vi "AM Measurement Compensation.vi"(11 "Mean Data in":dbl[](array[numeric])) -> (3 "Mean Data Compensated out":dbl[](array[numeric]))   [LabVIEW 2020, in "Motion.lvlib"]
uses:
  Motion.lvlib
  support/PCT FGV CMD.ctl
  Test Driver/Test Driver.lvlib
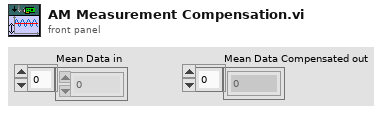
[diagram p1: front panel]
types:
  T1 = typedef "PCT FGV CMD.ctl" = enum16{"INIT", "GET", "SET"}
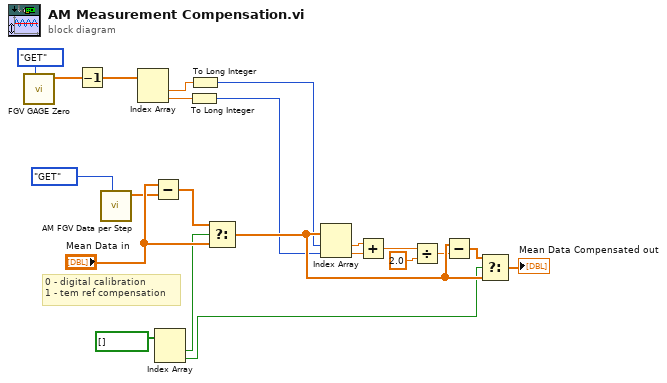
[diagram p0: block diagram]
diagram:
  # "0 - digital calibration\n1 - tem ref compensation"
  n1 = call "FGV GAGE Zero.vi"("CMD"=PCT_FGV_CMD."GET") -> ("output"=w12:dbl[])  [unwired: 9 in, 1 out]
  n2 = Decrement(x=w12) -> (x-1=w2:dbl[])
  n3 = call "AM FGV Data per Step.vi"("CMD"=PCT_FGV_CMD."GET") -> ("All Data out"=w13:dbl[])  [unwired: 9 in, 1 out]
  n4 = Index Array(array=w2) -> (element #1=w17:dbl, element #2=w9:dbl)  [unwired: 2 in]
  n5 = Subtract(x="Mean Data in", y=w13) -> (x-y=w15:dbl[])
  n6 = Index Array(array=bool[] [] ("Status Out")) -> (element #1=w14:bool, element #2=w19:bool)  [unwired: 2 in]
  n7 = To Long Integer(number=w9) -> (32bit integer=w8:i32)
  n8 = To Long Integer(number=w17) -> (32bit integer=w18:i32)
  n9 = Select(t=w15, s=w14, f="Mean Data in") -> (s? t:f=w21:dbl[])
  n10 = Index Array(array=w21, index #1=w18, index #2=w8) -> (element #1=w7:dbl, element #2=w6:dbl)
  n11 = Add(x=w7, y=w6) -> (x+y=w5:dbl)
  n12 = Divide(x=w5, y=2.0) -> (x/y=w3:dbl)
  n13 = Subtract(x=w21, y=w3) -> (x-y=w20:dbl[])
  n14 = Select(t=w20, s=w19, f=w21) -> (s? t:f=→"Mean Data Compensated out":dbl[])
